vi "UnitTest_UpdateData.vi"(8 "error in (no error)":errorcluster) -> (0 "error out":errorcluster)   [LabVIEW 2014, in "TableLogger_SQLite_Actor.lvlib" / "TableLogger_SQLite_Actor.lvclass"]
uses:
  TableLogger_SQLite_Actor.lvclass
  TableLogger_Actor/TableLoggerConfig.ctl
  TableLogger_Actor/TableLoggerTypes.ctl
  TableLogger_Actor/TableLoggerBackupConfig.ctl
  <vilib>/addons/_JKI Toolkits/Caraya/classes/Assert/Assert.lvclass
  <vilib>/addons/_JKI Toolkits/Caraya/classes/Test/Test.lvclass
  TableLogger_Actor/TableLogger_Actor.lvlib
panel:
  # "Please See the BlockDiagram for Update - Unit Test"
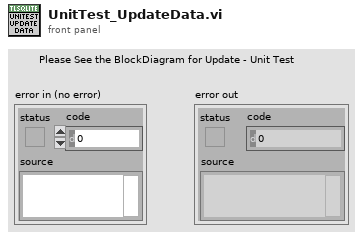
[diagram p1: front panel]
types:
  T1 = typedef "TableLogger_Actor.lvlib/TableLoggerConfig.ctl" = cluster{"TableLogger":T2, "DB File Path":path, "DB Backup Config":T3}
  T2 = typedef "TableLogger_Actor.lvlib/TableLoggerTypes.ctl" = enum16{"CSV Logger", "SQLite Logger"}
  T3 = typedef "TableLogger_Actor.lvlib/TableLoggerBackupConfig.ctl" = cluster{"Directory":path, "UTC Time Format":bool, "On Launch":bool, "Interval (Hours)":dbl, "Size Multiples (Bytes)":i32}
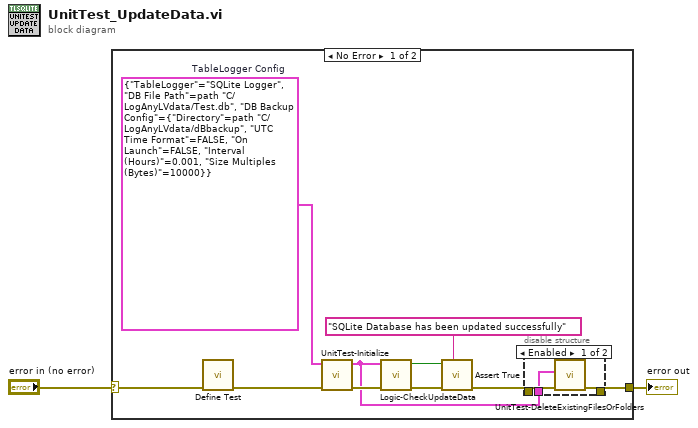
[diagram p0: block diagram]
diagram:
  n1 = case shown="No Error" "error in (no error)" {
    selector: "error in (no error)" -> [w11 w16]
    tunnel: [w5 w16] -> w2
    frame No Error {
      w4 = T1 {"TableLogger"=enum."SQLite Logger", "DB File Path"=path "C:/LogAnyLVdata/Test.db", "DB Backup Config"={"Directory"=path "C:/LogAnyLVdata/dBbackup", "UTC Time Format"=FALSE, "On Launch"=FALSE, "Interval (Hours)"=0.001, "Size Multiples (Bytes)"=10000}}  # TableLogger Config
      n2 = call <vilib>:"Define Test.vi"("error in (no error)"=w11) -> ("error out"=w8:errorcluster)  [unwired: 10 in]
      n3 = call "UnitTest-Initialize.vi"("error in"=w8, "Config IN"=w4) -> ("error out"=w7:errorcluster, "Config OUT"=w3:T1)  [unwired: 7 in, 1 out]
      n4 = call "Logic-CheckUpdateData.vi"("error in (no error)"=w7, "TableLogger Config"=w3) -> ("error out"=w10:errorcluster, "Update?T"=w9:bool)  [unwired: 8 in]
      n5 = call <vilib>:"Assert True.vi"("Label"="SQLite Database has been updated successfully", "error in (no error)"=w10, "True?"=w9) -> ("error out"=w6:errorcluster)  [unwired: 8 in]
      n6 = disable-structure shown="Enabled" {
        disable-tunnel: w6 -> [w15 _]
        disable-tunnel: [w14 _] -> w5
        disable-tunnel: w3 -> [w13 _]
        frame Enabled {
          n7 = call "UnitTest-DeleteExistingFilesOrFolders.vi"("error in (no error)"=w15, "Config IN"=w13) -> ("error out"=w14:errorcluster)  [unwired: 9 in]
        }
        frame Disabled {
        }
      }
    }
    frame Error {
    }
  }
  "error out" <- w2
